vi "NDMotor_SetTransmission.vi"(8 "error in":errorcluster, 10 "Laser Transmission (%)":i32, 11 "VISA resource name":refnum<visa-resource-name>) -> (0 "error out":errorcluster, 2 "ND Filter Position":i32, 3 "VISA resource name out":refnum<visa-resource-name>)   [LabVIEW 2024]
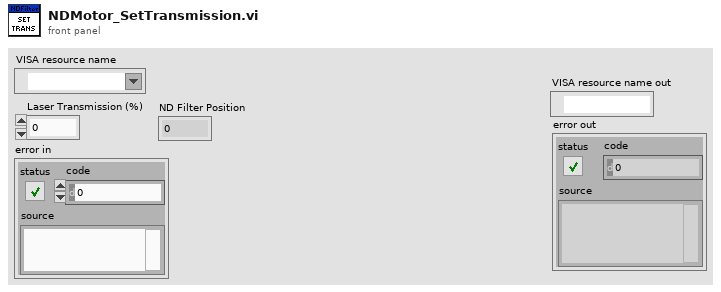
[diagram p1: front panel]
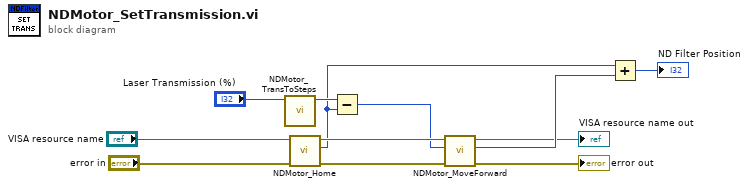
[diagram p0: block diagram]
diagram:
  n1 = call "NDMotor_TransToSteps.vi"("Transmission"="Laser Transmission (%)") -> ("Steps"=w11:i32)  [unwired: 10 in]
  n2 = call "NDMotor_Home.vi"("error in"="error in", "VISA resource name"="VISA resource name") -> ("error out"=w8:errorcluster, "home offset steps"=w3:i32, "VISA resource name out"=w9:refnum<visa-resource-name>)  [unwired: 6 in, 1 out]
  n3 = Subtract(x=w11, y=w3) -> (x-y=w4:i32)
  n4 = call "NDMotor_MoveForward.vi"("error in"=w8, "Steps"=w4, "VISA resource name"=w9) -> ("error out"=→"error out":errorcluster, "steps"=w6:i32, "VISA resource name out"=→"VISA resource name out":refnum<visa-resource-name>)  [unwired: 5 in, 1 out]
  n5 = Add(x=w3, y=w6) -> (x+y=→"ND Filter Position":i32)
